vi "Read Processes.vi"(4 "Error In":errorcluster, 6 "Launch Condition":T1, 7 "Config Data in":refnum<class "Config Data.lvclass">) -> (0 "Error Out":errorcluster, 2 "Processes to Launch":T2[](array[typedef]), 3 "Config Data out":refnum<class "Config Data.lvclass">)   [LabVIEW 2020, in "Config Data.lvlib" / "Config Data.lvclass"]
uses:
  Config Data.lvclass
  typedefs/Process Launch Data.ctl
  typedefs/Process Type.ctl
  typedefs/Launch Location.ctl
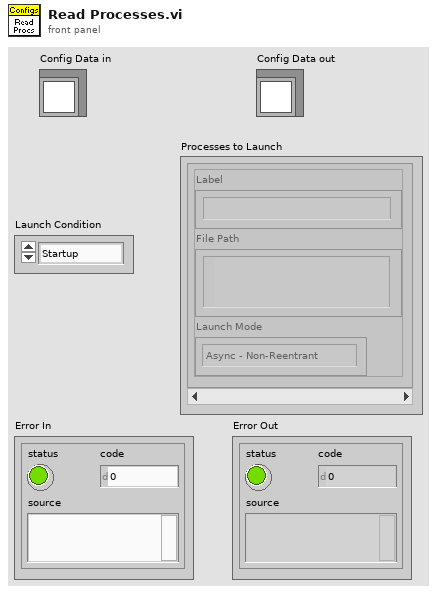
[diagram p1: front panel]
types:
  T1 = typedef "Config Data.lvlib/Config Data.lvclass/Launch Location.ctl" = enum16{"Startup", "Subpanels"}
  T2 = typedef "Config Data.lvlib/Config Data.lvclass/Process Launch Data.ctl" = cluster{"Label":string, "File Path":path, "Launch Mode":T3}
  T3 = typedef "Config Data.lvlib/Config Data.lvclass/Process Type.ctl" = enum16{"Async - Non-Reentrant", "Async - Reentrant", "Run Method - Non-Reentrant", "Run Method - Reentrant"}
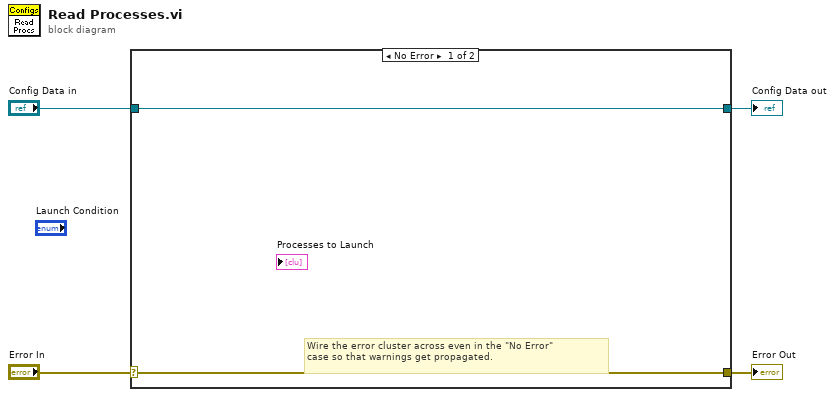
[diagram p0: block diagram]
diagram:
  n1 = case shown="No Error" "Error In" {
    selector: "Error In" -> [w5 w8]
    tunnel: [w5 w8] -> w3
    tunnel: [w6 w7] -> w1
    tunnel: "Config Data in" -> [w6 w7]
    frame No Error {
      # "Wire the error cluster across even in the \"No Error\"\ncase so that warnings get propagated."
    }
    frame Error {
    }
  }
  "Error Out" <- w3
  "Config Data out" <- w1
